vi "CreateCore.vi"(8 "error in (no error)":errorcluster, 10 "ParamsArray":variant[](array[variant]), 11 "Creator in":refnum<class "Creator.lvclass">) -> (0 "error out":errorcluster, 3 "Creator out":refnum<class "Creator.lvclass">)   [LabVIEW 2020, in "FactoryMethod.lvlib" / "Creator.lvclass"]
uses:
  Creator.lvclass
  Private/TypeDef/privateData.ctl
  ConcreteCreatorB/Product/Product.lvclass
  Creator.lvclass/Creator.ctl
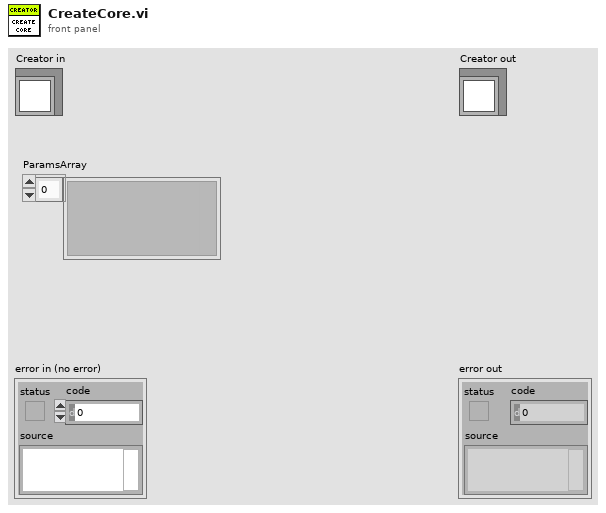
[diagram p1: front panel]
types:
  T1 = typedef "FactoryMethod.lvlib/Creator.lvclass/privateData.ctl" = cluster{"Product":refnum<class "Product.lvclass">}
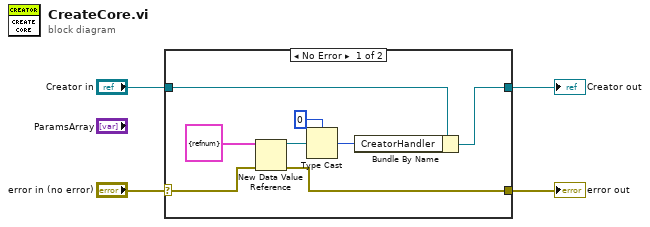
[diagram p0: block diagram]
diagram:
  n1 = case shown="No Error" "error in (no error)" {
    selector: "error in (no error)" -> [w6 w14]
    tunnel: [w7 w14] -> w1
    tunnel: [w9 w13] -> w3
    tunnel: "Creator in" -> [w8 w13]
    frame No Error {
      n2 = New Data Value Reference(data value=T1 {"Product"=refnum} ("privateData"), error in=w6) -> (data value reference=w12:refnum<data-value>, error out=w7:errorcluster)
      n3 = Type Cast(type=u32 0, x=w12) -> (*(type *) &x=w10:u32)
      n4 = Bundle By Name(cluster=w8, "CreatorHandler"=w10) -> (w9:refnum<class "Creator.lvclass">)
    }
    frame Error {
    }
  }
  "error out" <- w1
  "Creator out" <- w3
